vi "Creators Is Created Queue.vi"(10 "Created Queue Alias":string, 11 "Hello World Event in":refnum<class "Hello World Event.lvclass">) -> (2 "Is Created Queue?":bool, 3 "Hello World Event out":refnum<class "Hello World Event.lvclass">)   [LabVIEW 2021, in "Hello World Event.lvlib" / "Hello World Event.lvclass"]
uses:
  Hello World Event.lvclass
  Hello World Event.lvclass/Hello World Event.ctl
  <vilib>/Nathan Davis/jettl/jettl/Event/Event.lvclass
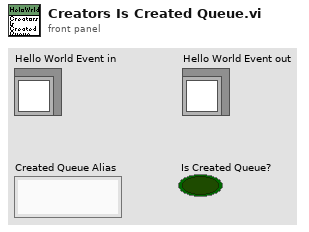
[diagram p1: front panel]
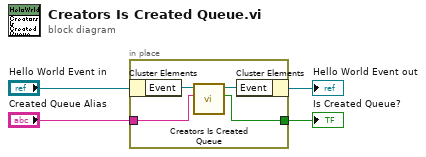
[diagram p0: block diagram]
diagram:
  n1 = in-place {
    in-place-border: [w6] -> w2
    in-place-border: "Created Queue Alias" -> [w5]
    n2 = in-place-cluster #1("Hello World Event in") -> ("Event"=w8:refnum<class "Event.lvclass">)
    n3 = call-dynamic "Creators Is Created Queue.vi"("Created Queue Alias"=w5, "Event in"=w8) -> ("Is Created Queue?"=w6:bool, "Event out"=w7:refnum<class "Event.lvclass">)  [unwired: 8 in]
    n4 = in-place-cluster #1("Event"=w7) -> (→"Hello World Event out":refnum<class "Hello World Event.lvclass">)
  }
  "Is Created Queue?" <- w2
